vi "Test Configuration File Creates non existing Folder Structure.vi"(8 "error in (no error)":errorcluster, 11 "Process Test In":refnum<class "Configuration File Process Interface Test.lvclass">) -> (0 "error out":errorcluster, 3 "Process Test Out":refnum<class "Configuration File Process Interface Test.lvclass">)   [LabVIEW 2020, in "Configuration File Process Interface Test.lvclass"]
uses:
  Configuration File Process Interface Test.lvclass
  C:/Program Files (x86)/National Instruments/LabVIEW 2020/vi.lib/Astemes/LUnit/Test Case.lvclass
  Mock Configurable Process/Mock Configurable Process.lvclass
  <vilib>/Astemes/LUnit/Test Case.lvclass/Test Case.ctl
  <vilib>/Astemes/LUnit/Palette/Fail.vi
  <vilib>/Astemes/LUnit/Palette/Pass.vi
  <vilib>/Astemes/LUnit/Set Assertion Type.vi
  <vilib>/Astemes/LUnit/Add test result.vi
  <vilib>/Astemes/LUnit/LUnit Record Assertion Result.vi
  <vilib>/Astemes/LUnit/LUnit Aggregate Assertion Results.vi
  <vilib>/Astemes/LUnit/Method Result/LUnit Merge Status.vi
  <vilib>/Astemes/LUnit/LUnit Concatenate result strings.vi
  <vilib>/Astemes/LUnit/Test Case.lvclass
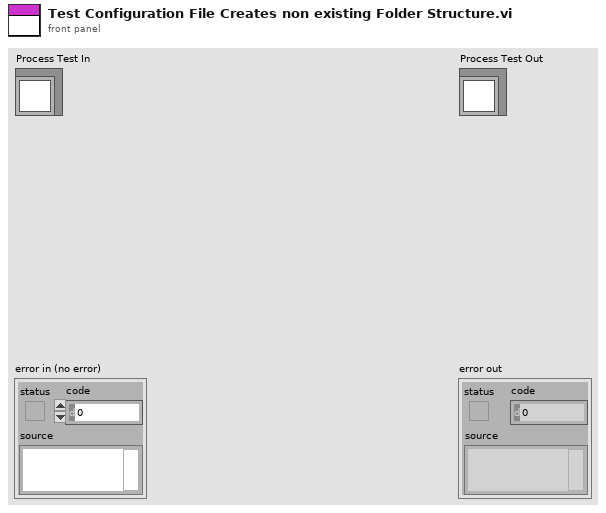
[diagram p1: front panel]
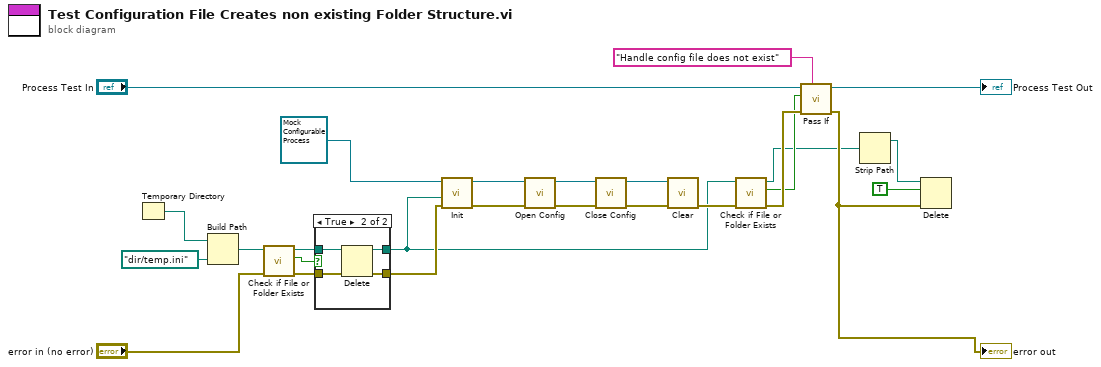
[diagram p0: block diagram]
diagram:
  n1 = Temporary Directory() -> (w21:path)
  n2 = Build Path(base path=w21, name or relative path=path "dir/temp.ini") -> (appended path=w19:path)
  n3 = call <vilib>:"Check if File or Folder Exists.vi"("error in (no error)"="error in (no error)", "path"=w19) -> ("error out"=w14:errorcluster, "file or folder exists?"=w11:bool, "dup path"=w15:path)  [unwired: 7 in]
  n4 = case shown="True" w11 {
    tunnel: w15 -> [w28 w32]
    tunnel: [w28 w31] -> w8
    tunnel: w14 -> [w27 w30]
    tunnel: [w27 w29] -> w12
    frame False {
    }
    frame True {
      n5 = Delete(path (use dialog)=w32, error in=w30) -> (deleted path=w31:path, error out=w29:errorcluster)  [unwired: 3 in, 1 out]
    }
  }
  n6 = call-dynamic "Init.vi"("error in (no error)"=w12, "Config File Path"=w8, "Process In"=refnum<class "Mock Configurable Process.lvclass"> refnum ("Mock Configurable.lvclass")) -> ("error out"=w24:errorcluster, "Process Out"=w25:refnum<class "Mock Configurable Process.lvclass">)  [unwired: 7 in]
  n7 = call-dynamic "Open Config.vi"("error in (no error)"=w24, "Configuration File File In"=w25) -> ("error out"=w10:errorcluster, "Configuration File File Out"=w2:refnum<class "Mock Configurable Process.lvclass">)  [unwired: 8 in]
  n8 = call-dynamic "Close Config.vi"("error in (no error)"=w10, "Configuration File File In"=w2) -> ("error out"=w3:errorcluster, "Configuration File File Out"=w1:refnum<class "Mock Configurable Process.lvclass">)  [unwired: 8 in]
  n9 = call-dynamic "Clear.vi"("error in (no error)"=w3, "Process In"=w1) -> ("error out"=w18:errorcluster)  [unwired: 9 in]
  n10 = call <vilib>:"Check if File or Folder Exists.vi"("error in (no error)"=w18, "path"=w8) -> ("error out"=w17:errorcluster, "file or folder exists?"=w16:bool, "dup path"=w6:path)  [unwired: 7 in]
  n11 = call <vilib>:"Pass If.vi"("Description"="Handle config file does not exist", "error in (no error)"=w17, "Pass?"=w16, "LUnit Test Case In"="Process Test In") -> ("error out"=w9:errorcluster, "LUnit Test Case Out"=→"Process Test Out":refnum<class "Configuration File Process Interface Test.lvclass">)  [unwired: 6 in]
  "error out" <- w9
  n12 = Strip Path(path=w6) -> (stripped path=w7:path)  [unwired: 1 out]
  n13 = Delete(path (use dialog)=w7, entire hierarchy (F)=TRUE, error in=w9) -> ()  [unwired: 2 in, 3 out]
